vi "ni579x Initialize Characterization Data (5791).vi"(5 "Device Data Header":T4={"Checksum"=0, "Number of Channels"=168, "Number of Attenuations"=[], "Number of Attenuator Settings"=[], "Number of Gain Settings"=[], "Pointer to Cal Data"=[255, 128], "Number of Reserved Bytes"=7, "Number of Frequencies"=[64, 32]} {"Checksum" format="%x"}, 11 "Error In":errorcluster) -> (6 "Characterization Data":T1[](array[typedef]) {"Frequencies [Hz]" format="%#_6p"}, 15 "Error Out":errorcluster)   [LabVIEW 2015, in "ni579x Config v2 Host.lvlib"]
uses:
  <instrlib>/ni579x/Config/v2/Host/ni579x Config v2 Host.lvlib
  <instrlib>/ni579x/Config/v2/Shared/Types/EEPROM/ni579x EEPROM Device Data Header.ctl
  <instrlib>/ni579x/Config/v2/Shared/Types/ni579x Characterization Data.ctl
  <instrlib>/ni579x/Config/v2/Shared/Types/ni579x IQ Imbalance.ctl
  <instrlib>/ni579x/Config/v2/Shared/Types/ni579x Gain to Attenuation Mapping.ctl
  <instrlib>/ni579x/Config/v2/Shared/ni579x Config v2 Shared.lvlib
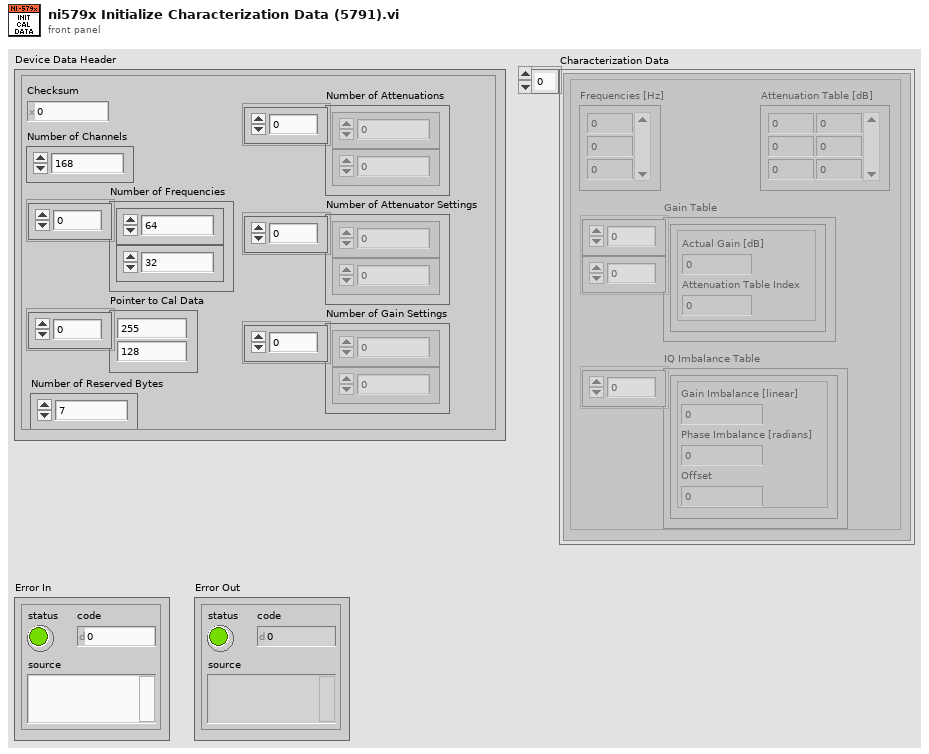
[diagram p1: front panel]
types:
  T1 = typedef "ni579x Config v2 Shared.lvlib/ni579x Characterization Data.ctl" = cluster{"Attenuation Table [dB]":dbl[][], "Frequencies [Hz]":dbl[], "IQ Imbalance Table":T2[], "Gain Table":T3[][]}
  T2 = typedef "ni579x Config v2 Shared.lvlib/ni579x IQ Imbalance.ctl" = cluster{"Gain Imbalance [linear]":dbl, "Phase Imbalance [radians]":dbl, "Offset":cdb}
  T3 = typedef "ni579x Config v2 Shared.lvlib/ni579x Gain to Attenuation Mapping.ctl" = cluster{"Actual Gain [dB]":dbl, "Attenuation Table Index":i32}
  T4 = typedef "ni579x Config v2 Shared.lvlib/ni579x EEPROM Device Data Header.ctl" = cluster{"Checksum":u32, "Number of Channels":u8, "Number of Attenuations":u16[], "Number of Attenuator Settings":u8[], "Number of Gain Settings":u8[], "Pointer to Cal Data":u32[], "Number of Reserved Bytes":i32, "Number of Frequencies":u16[]}
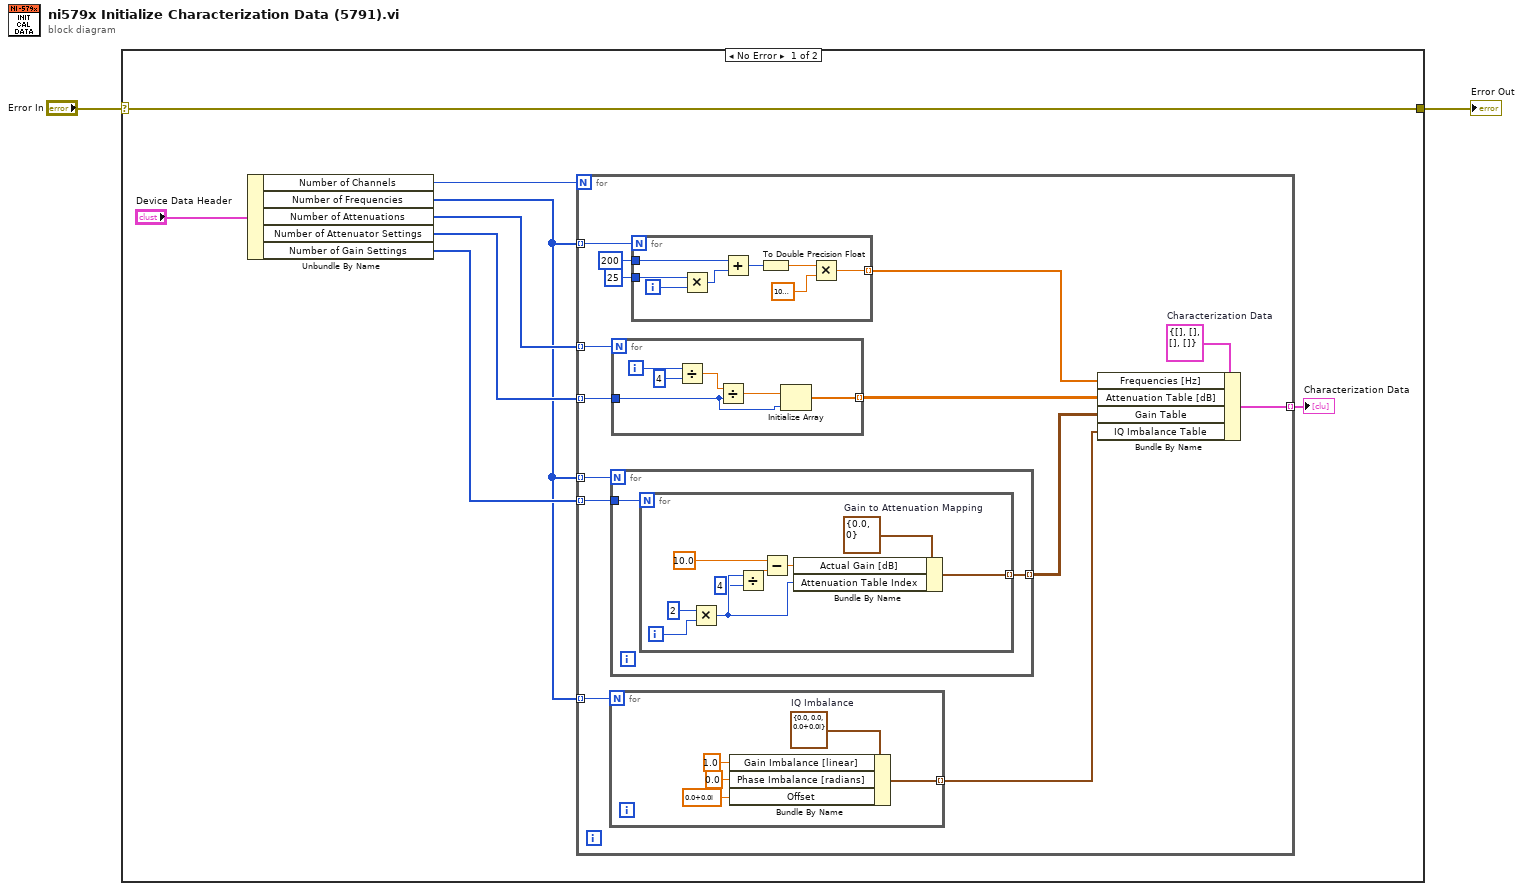
[diagram p0: block diagram]
diagram:
  n1 = case shown="No Error" "Error In" {
    selector: "Error In" -> [w5 w55]
    tunnel: [w5 w55] -> w1
    frame No Error {
      n2 = Unbundle By Name("Device Data Header") -> ("Number of Channels"=w4:u8, "Number of Frequencies"=w3:u16[], "Number of Attenuations"=w9:u16[], "Number of Attenuator Settings"=w8:u8[], "Number of Gain Settings"=w7:u8[])
      n3 = for {
        N: w4 -> [_]
        tunnel: w9 -> [w24] mode=indexing
        tunnel: w8 -> [w23] mode=indexing
        tunnel: w3 -> [w22] mode=indexing
        tunnel: w7 -> [w21] mode=indexing
        tunnel: w3 -> [w20] mode=indexing
        tunnel: [w15] -> w6 mode=indexing
        tunnel: w3 -> [w13] mode=indexing
        w19 = T1 {"Attenuation Table [dB]"=[], "Frequencies [Hz]"=[], "IQ Imbalance Table"=[], "Gain Table"=[]}  # Characterization Data
        n4 = for {
          N: w20 -> [_]
          tunnel: [w33] -> w16 mode=indexing
          w37 = T2 {"Gain Imbalance [linear]"=0.0, "Phase Imbalance [radians]"=0.0, "Offset"=0.0+0.0i}  # IQ Imbalance
          n5 = Bundle By Name(cluster=w37, "Gain Imbalance [linear]"=1.0, "Phase Imbalance [radians]"=0.0, "Offset"=cdb 0.0+0.0i) -> (w33:T2)
        }
        n6 = for {
          N: w22 -> [_]
          tunnel: w21 -> [w39]
          tunnel: [w38] -> w17 mode=indexing
          n7 = for {
            N: w39 -> [_]
            tunnel: [w43] -> w38 mode=indexing
            i -> [w44]
            w47 = T3 {"Actual Gain [dB]"=0.0, "Attenuation Table Index"=0}  # Gain to Attenuation Mapping
            n8 = Multiply(x=2, y=w44) -> (x*y=w41:i32)
            n9 = Divide(x=w41, y=4) -> (x/y=w42:dbl)
            n10 = Subtract(x=10.0, y=w42) -> (x-y=w46:dbl)
            n11 = Bundle By Name(cluster=w47, "Actual Gain [dB]"=w46, "Attenuation Table Index"=w41) -> (w43:T3)
          }
        }
        n12 = for {
          N: w24 -> [_]
          tunnel: w23 -> [w50]
          tunnel: [w49] -> w18 mode=indexing
          i -> [w54]
          n13 = Divide(x=w54, y=4) -> (x/y=w52:dbl)
          n14 = Divide(x=w52, y=w50) -> (x/y=w51:dbl)
          n15 = Initialize Array(w51, w50) -> (w49:dbl[])
        }
        n16 = for {
          N: w13 -> [_]
          tunnel: u16 25 ("Frequency Step Size") -> [w32]
          tunnel: u16 200 ("Start Frequency") -> [w30]
          tunnel: [w25] -> w14 mode=indexing
          i -> [w31]
          n17 = Multiply(x=w32, y=w31) -> (x*y=w29:i32)
          n18 = Add(x=w30, y=w29) -> (x+y=w28:i32)
          n19 = To Double Precision Float(number=w28) -> (double precision float=w27:dbl)
          n20 = Multiply(x=w27, y=1000000.0) -> (x*y=w25:dbl)
        }
        n21 = Bundle By Name(cluster=w19, "Frequencies [Hz]"=w14, "Attenuation Table [dB]"=w18, "Gain Table"=w17, "IQ Imbalance Table"=w16) -> (w15:T1)
      }
      "Characterization Data" <- w6
    }
    frame Error {
    }
  }
  "Error Out" <- w1
